vi "Read Orig Positions.vi"(3 "Setup file string":string, 4 "Analysis Info cluster In":T1[](array[typedef]) {"Sync Delay Time (s)" format="%.4f"; "Sd Error in Variance" format="%.2f"; "Skew_u" format="%.2f"; "% u'/U" format="%.2f"; "Sd Error in Mean" format="%.2f"; "Kurt_u" format="%.2f"; "u^4" format="%.2f"; "u^3" format="%.2f"; "U" format="%.2f"; "u^2" format="%.2f"}, 5 "Array in":string[][](array[string])) -> (1 "Analysis Info cluster Out":T1[](array[typedef]) {"Sync Delay Time (s)" format="%.4f"; "Sd Error in Variance" format="%.2f"; "Skew_u" format="%.2f"; "% u'/U" format="%.2f"; "Sd Error in Mean" format="%.2f"; "Kurt_u" format="%.2f"; "u^4" format="%.2f"; "u^3" format="%.2f"; "U" format="%.2f"; "u^2" format="%.2f"})   [LabVIEW 2020]
uses:
  Controls/Inst_type.ctl
  Controls/Instrument_Array.ctl
  Controls/Analysis_info_cluster.ctl
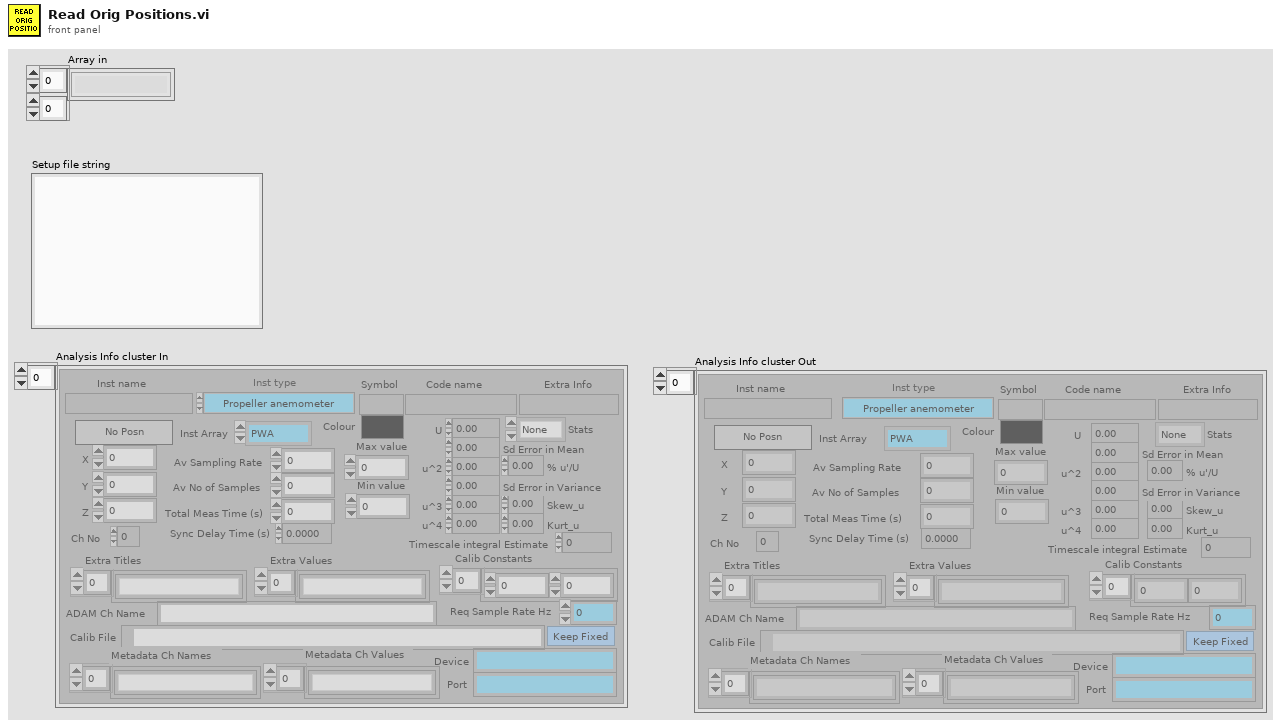
[diagram p1: front panel]
types:
  T1 = typedef "Analysis_info_cluster.ctl" = cluster{"Colour":u32, "Inst type":T2, "Inst name":string, "Symbol":string, "Code name":string, "Extra Info":string, "Inst Array":T3, "Extra Titles":string[], "Extra Values":string[], "U":dbl, "u^2":dbl, "u^3":dbl, "u^4":dbl, "Skew_u":dbl, "Kurt_u":dbl, "Sd Error in Mean":dbl, "% u'/U":dbl, "X":dbl, "Y":dbl, "Z":dbl, "Timescale integral Estimate":dbl, "Sd Error in Variance":dbl, "Calib File":path, "Calib Constants":dbl[], "Output Position":bool, "Stats":enum16{"None", "Basic", "Full"}, "Av Sampling Rate":dbl, "Av No of Samples":dbl, "Total Meas Time (s)":dbl, "ADAM Ch Name":string, "Max value":dbl, "Min value":dbl, "Req Sample Rate Hz":dbl, "Sync Delay Time (s)":dbl, "Ch No":i16, "Device":string, "Use Latest Calib":bool, "Port":string, "Metadata Ch Names":string[], "Metadata Ch Values":string[]}
  T2 = typedef "Inst_type.ctl" = enum16{"Propeller anemometer", "Raw voltage", "Pressure Transducer", "Pitot-static tube", "Preston tube", "Hot wire", "Cross wire 1", "Cross wire 2", "Generic Linear", "Generic Polynomial", "Generic BackPoly", "Fast FID", "Thermocouple", "Cold wire", "Pulsed Wire", "LDA Vel", "LDA Tran time", "LDA Arr time", "Microphone"}
  T3 = typedef "Instrument_Array.ctl" = enum16{"PWA", "LDA", "Analogue"}
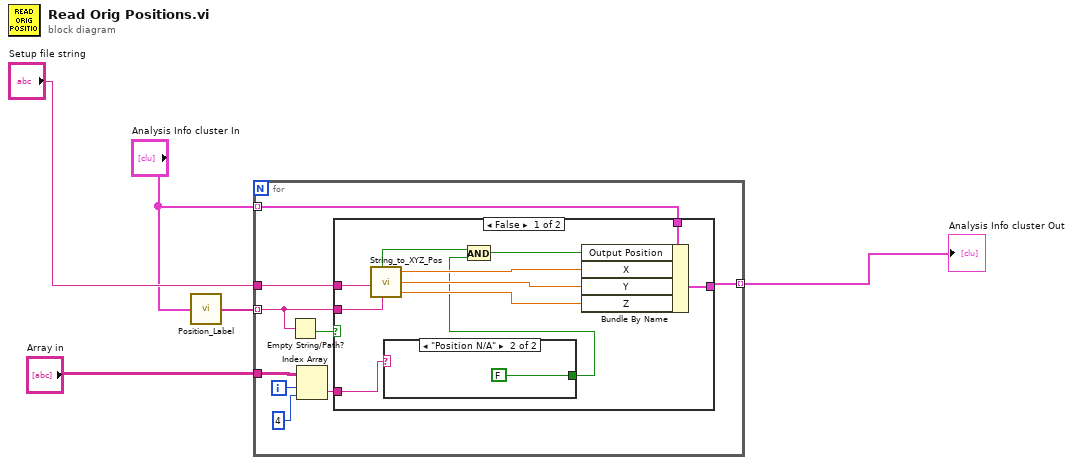
[diagram p0: block diagram]
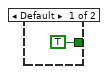
[diagram p2: hidden frame]
diagram:
  n1 = call "Position_Label.vi"("Analysis Info cluster"="Analysis Info cluster In") -> ("Position Label"=w2:string[])
  n2 = for {
    tunnel: "Analysis Info cluster In" -> [w13] mode=indexing
    tunnel: [w14] -> w4 mode=indexing
    tunnel: w2 -> [w11] mode=indexing
    tunnel: "Setup file string" -> [w12]
    tunnel: "Array in" -> [w9]
    i -> [w8]
    n3 = Empty String/Path?(string/path=w11) -> (empty?=w10:bool)
    n4 = Index Array(array=w9, index (row)=w8, index (col)=4 ("index")) -> (element=w6:string)
    n5 = case shown="False" w10 {
      tunnel: [w25 w28] -> w14
      tunnel: w13 -> [w24 w28]
      tunnel: w11 -> [w23 _]
      tunnel: w12 -> [w22 _]
      tunnel: w6 -> [w17 _]
      frame False {
        n6 = call "String_to_XYZ_Pos.vi"("Input string"=w22, "Position label"=w23) -> ("Some labels found"=w16:bool, "X"=w21:dbl, "Y"=w20:dbl, "Z"=w19:dbl)  [unwired: 2 in]
        n7 = case shown="\"Position N/A\"" w17 {
          tunnel: [TRUE FALSE] -> w15
          frame Default {
          }
          frame "Position N/A" {
          }
        }
        n8 = And(x=w16, y=w15) -> (x .and. y?=w18:bool)
        n9 = Bundle By Name(cluster=w24, "Output Position"=w18, "X"=w21, "Y"=w20, "Z"=w19) -> (w25:T1)
      }
      frame True {
      }
    }
  }
  "Analysis Info cluster Out" <- w4
